vi "make plots.vi"() -> ()   [LabVIEW 2016]
panel:
  in  "Numeric":i32=3
  out "fits 3":cluster{dbl[], dbl[]}[](graph)
  in  "fits 2":cluster{dbl[], dbl[]}[](graph)
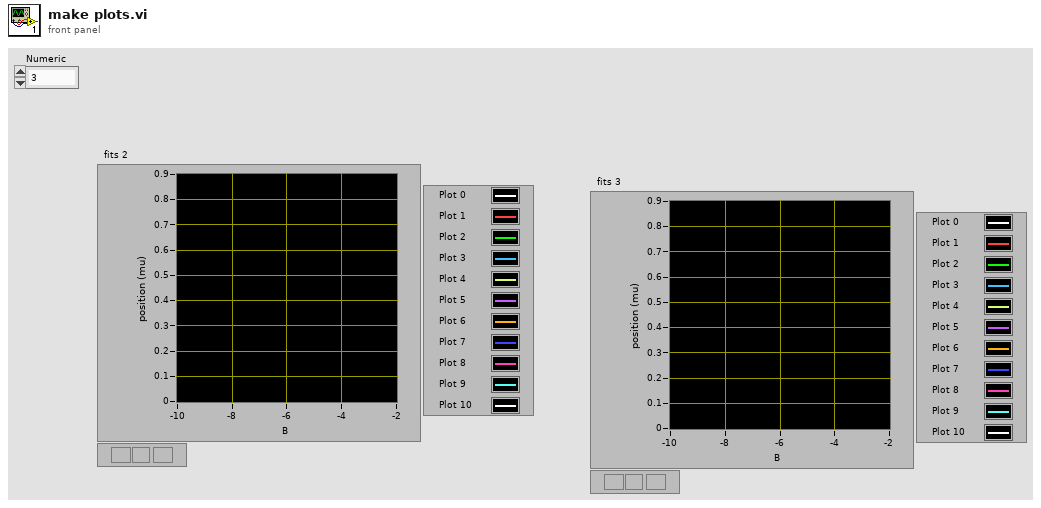
[diagram p1: front panel]
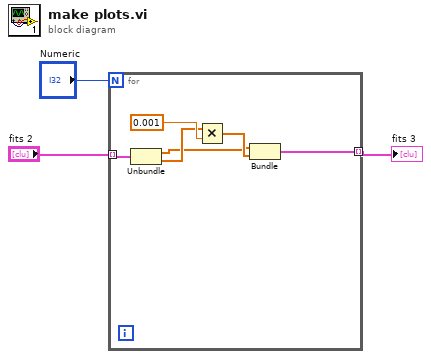
[diagram p0: block diagram]
diagram:
  n1 = for {
    N: "Numeric" -> [_]
    tunnel: "fits 2" -> [w9] mode=indexing
    tunnel: [w7] -> w2 mode=indexing
    n2 = Unbundle(w9) -> (w4:dbl[], w6:dbl[])
    n3 = Multiply(x=w6, y=0.001) -> (x*y=w5:dbl[])
    n4 = Bundle(w4, w5) -> (w7:cluster{dbl[], dbl[]})  [unwired: 1 in]
  }
  "fits 3" <- w2
